vi "Configure Color Sensor.vi"(0 "ColorSensorDevRef":T2={"I2CDevRef"={"DevStatus"={"status"=FALSE, "code"=0, "source"=""}, "Device Address"=0, "Handle"=0, "I2C Bus"=enum."Invalid"}} {"I2CDevRef"."Device Address" format="%.0x"}, 5 "ColorSensorResolution":T6, 7 "ColorSensorMeasurementRate":T5, 9 "GainFactor":T1, 11 "error in (no error)":errorcluster) -> (4 "ColorSensorDevRef out":T2={"I2CDevRef"={"DevStatus"={"status"=FALSE, "code"=0, "source"=""}, "Device Address"=0, "Handle"=0, "I2C Bus"=enum."Invalid"}} {"I2CDevRef"."Device Address" format="%.0x"}, 15 "error out":errorcluster)   [LabVIEW 2018, in "ColorSensor.lvlib"]
uses:
  ColorSensor.lvlib
  ColorSensorDevRef.ctl
  <vilib>/Rock Robotics/WPI/I2C/WPI_I2CDevRef.ctl
  <vilib>/Rock Robotics/SystemInterfaces/i2clib/i2c_bus.ctl
  ColorSensorResolution.ctl
  ColorSensorMeasurementRate.ctl
  GainFactor.ctl
  Registers.ctl
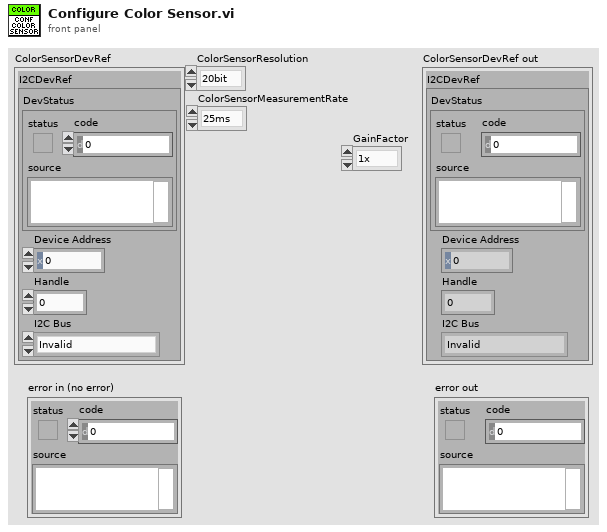
[diagram p1: front panel]
types:
  T1 = typedef "ColorSensor.lvlib/GainFactor.ctl" = enum16{"1x", "3x", "6x", "9x", "18x"}
  T2 = typedef "ColorSensor.lvlib/ColorSensorDevRef.ctl" = cluster{"I2CDevRef":T3}
  T3 = typedef "WPI_I2CDevRef.ctl" = cluster{"DevStatus":errorcluster, "Device Address":u8, "Handle":i32, "I2C Bus":T4}
  T4 = typedef "i2c_bus.ctl" = enum16{"I2C On-Board", "I2C MXP", "Invalid"}
  T5 = typedef "ColorSensor.lvlib/ColorSensorMeasurementRate.ctl" = enum16{"25ms", "50ms", "100ms", "200ms", "500ms", "1000ms", "2000ms"}
  T6 = typedef "ColorSensor.lvlib/ColorSensorResolution.ctl" = enum16{"20bit", "19bit", "18bit", "17bit", "16bit", "13bit"}
  T7 = typedef "ColorSensor.lvlib/Registers.ctl" = enum16{"MainCtrl", "ProximitSensorLED", "ProximitySensorPulse", "ProximitySensorRate", "LightSensorMeasurementRate", "LightSensorGainRegister", "PartIDRegister", "MainStatus", "ProximityData", "ProximityData1", "InfraredData", "InfraredData1", "InfraredData2", "GreenData", "GreenData1", "GreenData2", "BlueData", "BlueData1", "BlueData2", "RedData", "RedData1", "RedData2"}
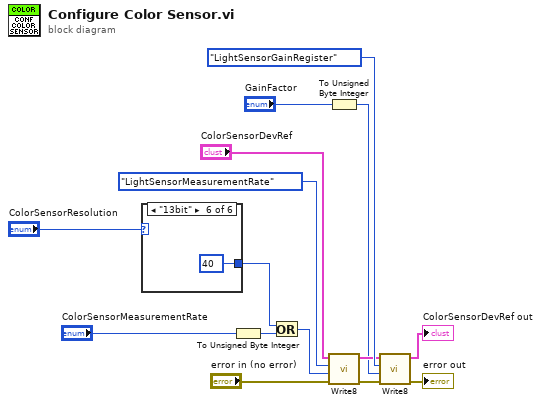
[diagram p0: block diagram]
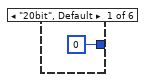
[diagram p2: hidden frame]
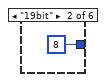
[diagram p3: hidden frame]
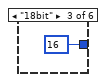
[diagram p4: hidden frame]
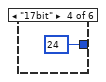
[diagram p5: hidden frame]
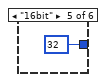
[diagram p6: hidden frame]
diagram:
  n1 = case shown="\"13bit\"" "ColorSensorResolution" {
    tunnel: [u8 0 ("Data") u8 8 ("Data") u8 16 ("Data") u8 24 ("Data") u8 32 ("Data") u8 40 ("Data")] -> w12
    frame "20bit", Default {
    }
    frame "19bit" {
    }
    frame "18bit" {
    }
    frame "17bit" {
    }
    frame "16bit" {
    }
    frame "13bit" {
    }
  }
  n2 = To Unsigned Byte Integer(number="ColorSensorMeasurementRate") -> (unsigned 8bit integer=w10:u8)
  n3 = Or(x=w12, y=w10) -> (x .or. y?=w9:u8)
  n4 = To Unsigned Byte Integer(number="GainFactor") -> (unsigned 8bit integer=w1:u8)
  n5 = call "Write8.vi"("error in (no error)"="error in (no error)", "Data"=w9, "Registers"=Registers."LightSensorMeasurementRate", "ColorSensorDevRef"="ColorSensorDevRef") -> ("error out"=w5:errorcluster, "ColorSensorDevRef out"=w6:T2)  [unwired: 6 in]
  n6 = call "Write8.vi"("error in (no error)"=w5, "Data"=w1, "Registers"=Registers."LightSensorGainRegister", "ColorSensorDevRef"=w6) -> ("error out"=→"error out":errorcluster, "ColorSensorDevRef out"=→"ColorSensorDevRef out":T2)  [unwired: 6 in]
